vi "Check_if_activated_drift(SubVI).vi"(7 "Override":bool, 9 "activate  every  iterations":i32, 10 "activated?":bool, 11 "Iteration":i32) -> (3 "perform action":bool)   [LabVIEW 2014]
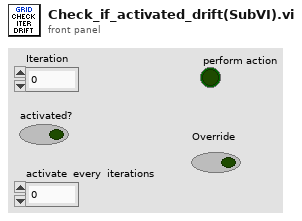
[diagram p1: front panel]
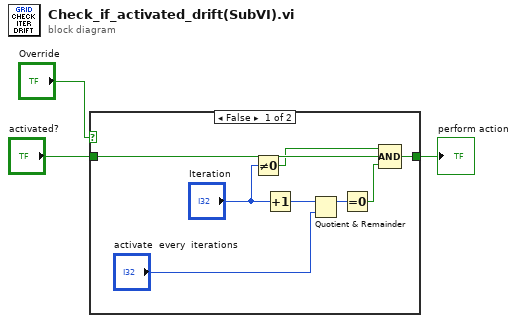
[diagram p0: block diagram]
diagram:
  n1 = case shown="False" "Override" {
    tunnel: "activated?" -> [w6 w12]
    tunnel: [w8 w12] -> w2
    frame False {
      n2 = Not Equal To 0?(x="Iteration") -> (x != 0?=w4:bool)
      n3 = Increment(x="Iteration") -> (x+1=w10:i32)
      n4 = Quotient & Remainder(x=w10, y="activate  every  iterations") -> (x-y*floor(x/y)=w9:i32)  [unwired: 1 out]
      n5 = Equal To 0?(x=w9) -> (x = 0?=w7:bool)
      n6 = Compound Arithmetic op=AND(w4, w6, w7) -> (w8:bool)
    }
    frame True {
    }
  }
  "perform action" <- w2
